vi "Day13-1.vi"() -> ()   [LabVIEW 2021]
panel:
  out "sum":i16
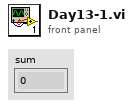
[diagram p1: front panel]
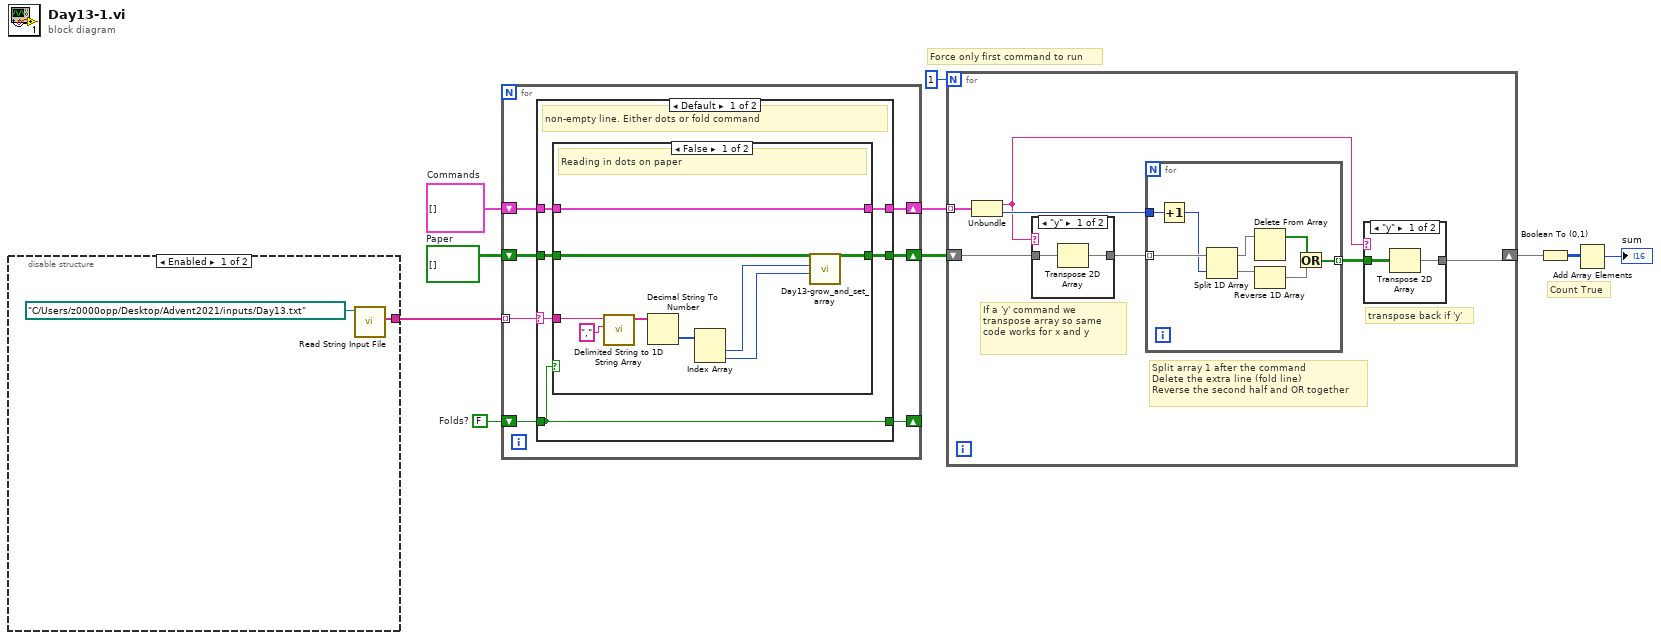
[diagram p0: block diagram]
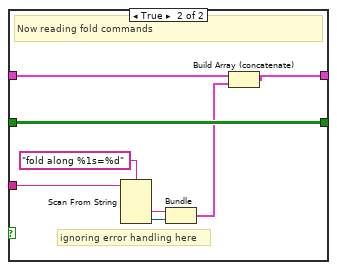
[diagram p4: hidden frame]
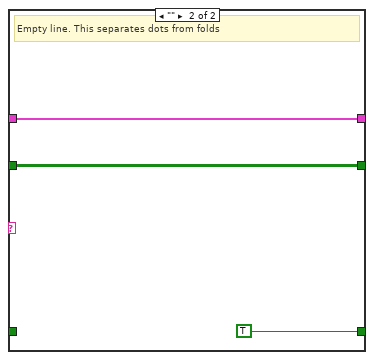
[diagram p5: hidden frame]
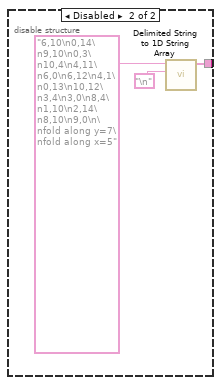
[diagram p6: hidden frame]
diagram:
  w7 = cluster{string, i32}[] []  # Commands
  w8 = bool[][] []  # Paper
  w9 = FALSE  # Folds?
  # "Force only first command to run"
  # "Count True"
  n1 = disable-structure shown="Enabled" {
    disable-tunnel: [w11 w13] -> w10
    frame Enabled {
      n2 = call "Read String Input File.vi"("file path (dialog if empty)"=path "C:/Users/z0000opp/Desktop/Advent2021/inputs/Day13.txt") -> ("input values"=w11:string[])  [unwired: 10 in]
    }
    frame Disabled {
      n3 = call <vilib>:"Delimited String to 1D String Array.vi"("delimiter"="\n", "delimited string"="6,10\n0,14\n9,10\n0,3\n10,4\n4,11\n6,0\n6,12\n4,1\n0,13\n10,12\n3,4\n3,0\n8,4\n1,10\n2,14\n8,10\n9,0\n\nfold along y=7\nfold along x=5") -> ("string array"=w13:string[])  [unwired: 9 in]
    }
  }
  n4 = for {
    tunnel: w10 -> [w22] mode=indexing
    shift-right: [w18] -> _
    shift-left: w9 -> [w21]
    shift-right: [w19] -> w5
    shift-left: w8 -> [w20]
    shift-right: [w16] -> w6
    shift-left: w7 -> [w17]
    n5 = case shown="Default" w22 {
      selector: w22 -> [w28 _]
      tunnel: w21 -> [w25 _]
      tunnel: w20 -> [w27 w48]
      tunnel: [w26 w48] -> w19
      tunnel: [w25 TRUE] -> w18
      tunnel: w17 -> [w24 w46]
      tunnel: [w23 w46] -> w16
      frame Default {
        # "non-empty line. Either dots or fold command"
        n6 = case shown="False" w25 {
          tunnel: w28 -> [w37 w43]
          tunnel: w27 -> [w33 w45]
          tunnel: [w30 w45] -> w26
          tunnel: w24 -> [w29 w40]
          tunnel: [w29 w38] -> w23
          frame False {
            # "Reading in dots on paper"
            n7 = call <vilib>:"Delimited String to 1D String Array.vi"("delimiter"=",", "delimited string"=w37) -> ("string array"=w35:string[])  [unwired: 9 in]
            n8 = Decimal String To Number(string=w35) -> (number=w34:i32[])  [unwired: 2 in, 1 out]
            n9 = Index Array(array=w34) -> (element #1=w32:i32, element #2=w31:i32)  [unwired: 2 in]
            n10 = call "Day13-grow_and_set_array.vi"("row"=w31, "column"=w32, "Array in"=w33) -> ("Array out"=w30:bool[][])  [unwired: 8 in]
          }
          frame True {
            # "ignoring error handling here"
            # "Now reading fold commands"
            n11 = Scan From String(format string="fold along %1s=%d", input string=w43) -> (output 1=w42:string, output 2=w41:i32)  [unwired: 4 in, 3 out]
            n12 = Bundle(w42, w41) -> (w39:cluster{string, i32})  [unwired: 1 in]
            n13 = Build Array (concatenate)(w40, w39) -> (w38:cluster{string, i32}[])
          }
        }
      }
      frame "" {
        # "Empty line. This separates dots from folds"
      }
    }
  }
  n14 = for {
    N: 1 -> [_]
    tunnel: w6 -> [w55] mode=indexing
    shift-right: [w50] -> w4
    shift-left: w5 -> [w54]
    # "Split array 1 after the command\nDelete the extra line (fold line)\nReverse the second half and OR together"
    # "transpose back if 'y'"
    # "If a 'y' command we transpose array so same code works for x and y"
    n15 = Unbundle(w55) -> (w49:string, w52:i32)
    n16 = case shown="\"y\"" w49 {
      tunnel: w54 -> [w68 w69]
      tunnel: [w67 w69] -> w53
      frame "y" {
        n17 = Transpose 2D Array(2D array=w68) -> (transposed array=w67:bool[][])
      }
      frame "x", Default {
      }
    }
    n18 = for {
      tunnel: w53 -> [w66] mode=indexing
      tunnel: w52 -> [w65]
      tunnel: [w59] -> w51 mode=indexing
      n19 = Increment(x=w65) -> (x+1=w64:i32)
      n20 = Split 1D Array(array=w66, index=w64) -> (first subarray=w63:bool[], second subarray=w62:bool[])
      n21 = Delete From Array(array=w63) -> (array with subset deleted=w60:bool[])  [unwired: 2 in, 1 out]
      n22 = Reverse 1D Array(array=w62) -> (reversed array=w61:bool[])
      n23 = Or(x=w60, y=w61) -> (x .or. y?=w59:bool[])
    }
    n24 = case shown="\"y\"" w49 {
      tunnel: w51 -> [w57 w58]
      tunnel: [w56 w58] -> w50
      frame "y" {
        n25 = Transpose 2D Array(2D array=w57) -> (transposed array=w56:bool[][])
      }
      frame "x", Default {
      }
    }
  }
  n26 = Boolean To (0,1)(Boolean=w4) -> (0, 1=w3:i16[][])
  n27 = Add Array Elements(numeric array=w3) -> (sum=→"sum":i16)
